vi "PH_ImageCoG_Plotter.get i attribute.vi"(0 "i ref in":refnum<vi>, 5 "error in (no error)":errorcluster) -> (14 "i ref out":refnum<vi>, 16 "i attribute":T1 {"Calibration"."Status" items=["no info", "off/false/out", "on/true/in", "Failure", "Alarm", "Status 1", "Status 2", "Status 3"]}, 19 "error out":errorcluster)   [LabVIEW 2014, in "PH_ImageCoG_Plotter.lvlib"]
doc: "Gets the i attribute data of an object.\n\nLicense Agreement for this software:\n\nCopyright (C)\nGesellschaft für Schwerionenforschung, GSI\nPlanckstr. 1\n64291 Darmstadt\nGermany\n\nContact: D.Beck@gsi.de \n\nThis program is free software; you can redistribute it and/or modify it under the terms of the GNU General Public License as published by the Free Software Foundation; either version 2 of the license, or (at your option) any later version.\n\nThis program is distributed in the hope that it will be useful, but WITHOUT ANY WARRANTY; without even the implied warranty of MERCHANTABILITY or FITNESS FOR A PARTICULAR PURPOSE. See the GNU General License for more details (http://www.gnu.org).\n\nGesellschaft für Schwerionenforschung, GSI\nPlanckstr. 1, 64291 Darmstadt, Germany\nFor all questions and ideas contact: M.Richter@gsi.de, H.Brand@gsi.de or D.Beck@gsi.de.\nLast update: 17-JUN-2004"
uses:
  PH_ImageCoG_Plotter.lvlib
  PH_ImageCoG_Plotter.i attribute.ctl
  PH_ImageCalibrator/PH_ImageCalibrator.Calibration Data.ctl
  PH_StatusHandler/PH_StatusHandler.Status.ctl
  CSCore/BaseProcess/BaseProcess.event definition.ctl
  CSCore/CAEObj/CAEObj.event definition.ctl
  CSCore/BaseProcess/BaseProcess.descriptor string definition.ctl
  <vilib>/vision/Image Controls.llb/IMAQ Image.ctl
  CSCore/CAEObj/CAEObj.lvlib
  CSCore/BaseProcess/BaseProcess.lvlib
  PH_ImageCalibrator/PH_ImageCalibrator.lvlib
  PH_StatusHandler/PH_StatusHandler.lvlib
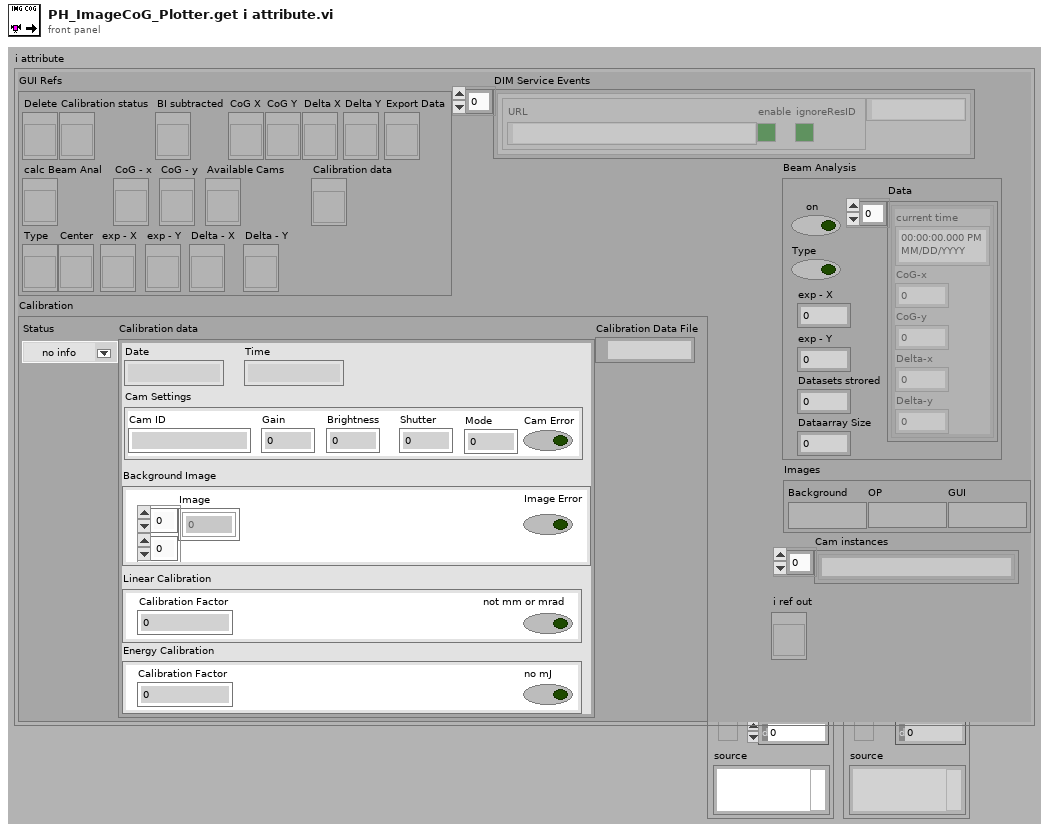
[diagram p1: front panel]
types:
  T1 = typedef "PH_ImageCoG_Plotter.lvlib/PH_ImageCoG_Plotter.i attribute.ctl" = cluster{"GUI Refs":cluster{"Delete":refnum<vi>, "Calibration status":refnum<vi>, "BI subtracted":refnum<vi>, "calc Beam Anal":refnum<vi>, "CoG - x":refnum<vi>, "CoG - y":refnum<vi>, "Type":refnum<vi>, "Center":refnum<vi>, "exp - X":refnum<vi>, "exp - Y":refnum<vi>, "Delta - X":refnum<vi>, "Delta - Y":refnum<vi>, "Available Cams":refnum<vi>, "CoG X":refnum<vi>, "CoG Y":refnum<vi>, "Delta X":refnum<vi>, "Delta Y":refnum<vi>, "Export Data":refnum<vi>, "Calibration data":refnum<vi>}, "Calibration":cluster{"Status":T2, "Calibration data":T3, "Calibration Data File":path}, "Beam Analysis":cluster{"on":bool, "exp - X":i32, "exp - Y":i32, "Type":bool, "Data":cluster{"current time":timestamp, "CoG-x":dbl, "CoG-y":dbl, "Delta-x":dbl, "Delta-y":dbl}[], "Datasets strored":i32, "Dataarray Size":i32}, "Cam instances":string[], "DIM Service Events":T4[], "Images":cluster{"Background":T7, "OP":T7, "GUI":T7}}
  T2 = typedef "PH_StatusHandler.lvlib/PH_StatusHandler.Status.ctl" = i16
  T3 = typedef "PH_ImageCalibrator.lvlib/PH_ImageCalibrator.Calibration Data.ctl" = cluster{"Date":string, "Time":string, "Cam Settings":cluster{"Cam ID":string, "Gain":dbl, "Brightness":dbl, "Shutter":dbl, "Cam Error":bool, "Mode":i32}, "Background Image":cluster{"Image":dbl[][], "Image Error":bool}, "Linear Calibration":cluster{"Calibration Factor":dbl, "not mm or mrad":bool}, "Energy Calibration":cluster{"Calibration Factor":dbl, "no mJ":bool}}
  T4 = typedef "BaseProcess.lvlib/BaseProcess.event definition.ctl" = cluster{"CAEEvtDef":T5, "Data Descriptor":T6}
  T5 = typedef "CAEObj.lvlib/CAEObj.event definition.ctl" = cluster{"URL":string, "enable":bool, "ignoreResID":bool}
  T6 = typedef "BaseProcess.lvlib/BaseProcess.descriptor string definition.ctl" = string
  T7 = typedef "IMAQ Image.ctl" = refnum<image>
  T8 = enum16{"SetAttribute", "GetAttribute", "CreateAttribute", "DestroyAttribute", "DestroyAllAtributes"}
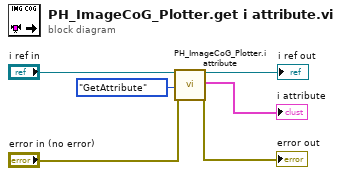
[diagram p0: block diagram]
diagram:
  n1 = call "PH_ImageCoG_Plotter.i attribute.vi"("VI Refnum"="i ref in", "Action"=T8."GetAttribute", "error in (no error)"="error in (no error)") -> ("VI Refnum out"=→"i ref out":refnum<vi>, "CLASS.i attribute out"=→"i attribute":T1, "error out"=→"error out":errorcluster)  [unwired: 14 in]
